vi "Publisher Do.vi"(8 "error in (no error)":errorcluster, 10 "Publisher in":refnum<class "Publisher.lvclass">, 11 "Publisher Msg in":refnum<class "Publisher Msg.lvclass">) -> (0 "error out":errorcluster, 2 "Publisher out":refnum<class "Publisher.lvclass">)   [LabVIEW 2020, in "Publisher.lvlib" / "Publisher Msg.lvclass"]
doc: "Execute an action on the Publisher.\nThe defautl implementation is empty."
uses:
  Publisher Msg.lvclass
  Publisher/Publisher.lvclass
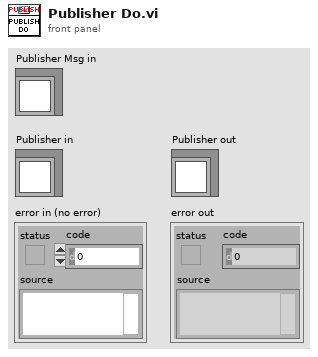
[diagram p1: front panel]
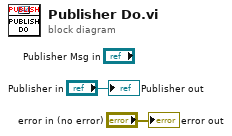
[diagram p0: block diagram]
diagram:
  "error out" <- "error in (no error)"
  "Publisher out" <- "Publisher in"
